vi "ADAM_Global.vi"() -> ()   [LabVIEW 2012]
uses:
  ADAM Client/Sub VIs/ADAM Controls/Update_scan_value.ctl
  ADAM Client/Sub VIs/ADAM Controls/Ch_description_ADAM.ctl
  ADAM Client/Sub VIs/ADAM Controls/Module_type_ADAM.ctl
  ADAM Client/Sub VIs/ADAM Controls/Function_ADAM.ctl
  ADAM Client/Sub VIs/ADAM Controls/Channel_State.ctl
  ADAM Client/Sub VIs/ADAM Controls/Calib_type_ADAM.ctl
  ADAM Client/Sub VIs/ADAM Controls/Address.ctl
  ADAM Client/Sub VIs/ADAM Controls/Client_State_Cluster.ctl
  ADAM Client/Sub VIs/ADAM Controls/Traverse_Level_State.ctl
  ADAM Client/Sub VIs/ADAM Controls/Comments_cluster.ctl
  ADAM Client/Sub VIs/ADAM Controls/Server_Control.ctl
  Sub VI's/ADAM_Comparitor.ctl
panel:
  in  "Comparitor Array":T1[](array[typedef])
  in  "Network Last checked":dbl
  out "All Ch names":string[](array[string])
  in  "Program Hung Clients":string[](array[string])
  in  "Server Control Array":T2[](array[typedef]) {"Default Value" format="%.2f"}
  in  "Comments Array":T3[](array[typedef])
  in  "Client State Array":T4[](array[typedef])
  in  "Update Ch Description Array":T6[](array[typedef]) {"Duty" format="%.0b"; "D" format="%#_5g"; "C" format="%#_5g"; "B" format="%#_5g"; "A" format="%#_5g"}
  in  "Update Current Value":T12[](array[typedef]) {"New Value" format="%.2f"}
  out "Active Ch Indicies":i32[](array[numeric])
  in  "2 Min average comment":string
  out "Scan comments":string[](array[string])
  in  "Current Channel Values":dbl[](array[numeric]) format="%.2f"
  out "Active Ch names":string[](array[string])
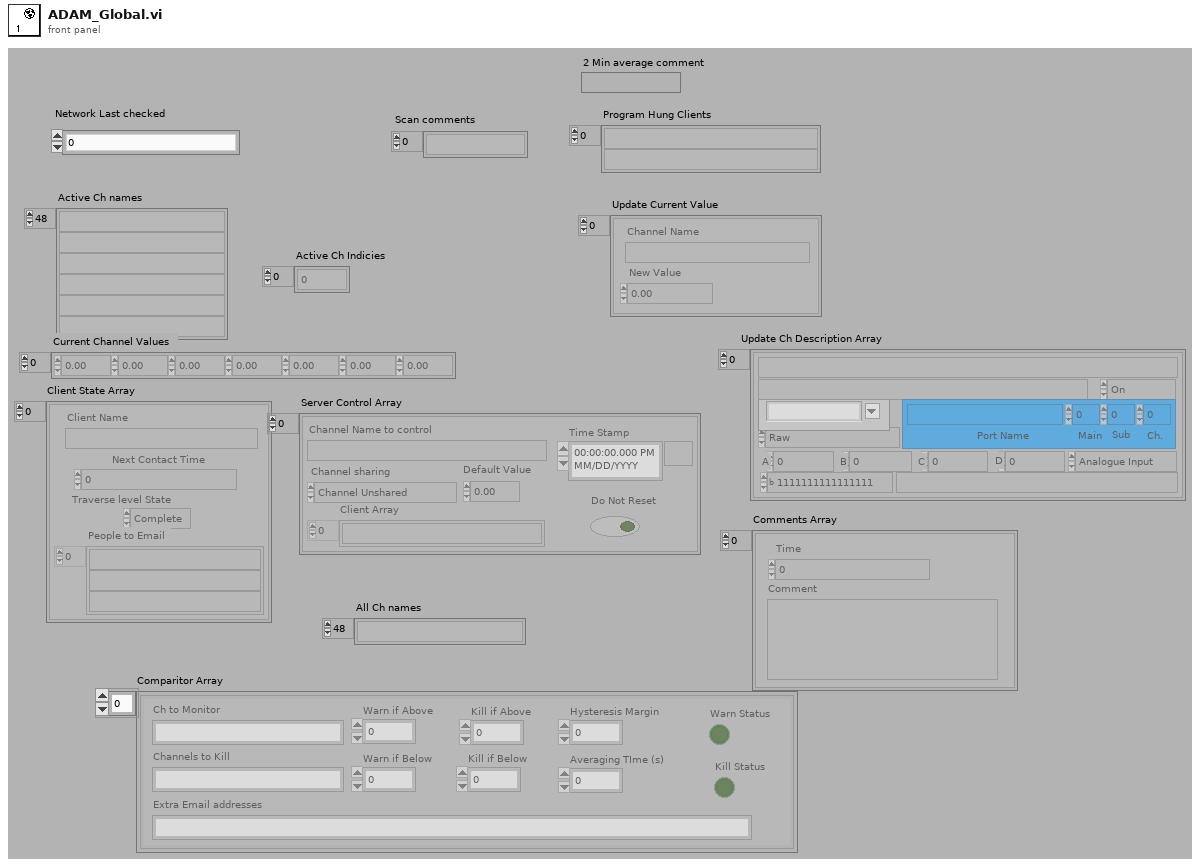
[diagram p1: front panel]
types:
  T1 = typedef "ADAM_Comparitor.ctl" = cluster{"Ch to Monitor":string, "Channels to Kill":string, "Warn if Above":dbl, "Warn if Below":dbl, "Kill if Above":dbl, "Kill if Below":dbl, "Hysteresis Margin":dbl, "Averaging TIme (s)":dbl, "Warn Status":bool, "Kill Status":bool, "Extra Email addresses":string}
  T2 = typedef "Server_Control.ctl" = cluster{"Channel Name to control":string, "Channel sharing":enum16{"Channel Unshared", "Channel Shared by Rig", "Channel Shared by Group"}, "Default Value":dbl, "Client Array":string[], "Time Stamp":timestamp, "Do Not Reset":bool}
  T3 = typedef "Comments_cluster.ctl" = cluster{"Time":dbl, "Comment":string}
  T4 = typedef "Client_State_Cluster.ctl" = cluster{"Client Name":string, "Traverse level State":T5, "People to Email":string[], "Next Contact Time":dbl}
  T5 = typedef "Traverse_Level_State.ctl" = enum16{"Running", "Complete"}
  T6 = typedef "Ch_description_ADAM.ctl" = cluster{"Ch Name":string, "Type":T7, "Function":T8, "Ch State":T9, "Calibration type":T10, "A":dbl, "B":dbl, "C":dbl, "D":dbl, "Comments":string, "Address":T11, "String":string, "Duty":u16}
  T7 = typedef "Module_type_ADAM.ctl" = string
  T8 = typedef "Function_ADAM.ctl" = enum16{"Analogue Input", "Digital Input", "Event counter", "Event rate", "Analogue Output", "Digital Output", "Relay Output"}
  T9 = typedef "Channel_State.ctl" = enum16{"On", "Off", "Always On", "Always Off"}
  T10 = typedef "Calib_type_ADAM.ctl" = enum16{"Raw", "Bx + A", "Cx^2 + Bx + A", "Dx^3 + Cx^2 + Bx + A", "In Band", "Hi-Tec Q", "Hi-Tec M_dot", "Text"}
  T11 = typedef "Address.ctl" = cluster{"Main":i32, "Ch.":i32, "Sub":i32, "Port Name":string}
  T12 = typedef "Update_scan_value.ctl" = cluster{"Channel Name":string, "New Value":dbl}
diagram:
